vi "VCS Get Device Name.vi"(8 "error in (no error)":errorcluster, 11 "axis in":cluster{"keyHandle":u32, "nodeId":u16}={"keyHandle"=0, "nodeId"=1}) -> (0 "error out":errorcluster, 2 "deviceName":string, 3 "axis out":cluster{"keyHandle":u32, "nodeId":u16}={"keyHandle"=0, "nodeId"=1})   [LabVIEW 2019]
doc: "<B>VCS Get Device Name</B> returns the device name to corresponding handle."
uses:
  Resources/EposCmd.dll
  Examples/maxonEPOS.lvlib
  Resources/EposCmd64.dll
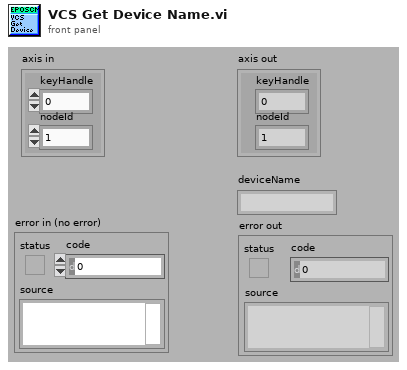
[diagram p1: front panel]
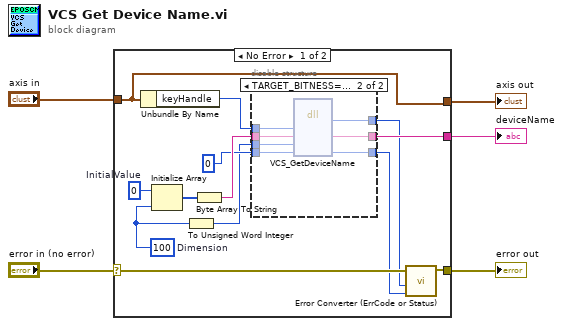
[diagram p0: block diagram]
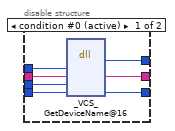
[diagram p2: hidden frame]
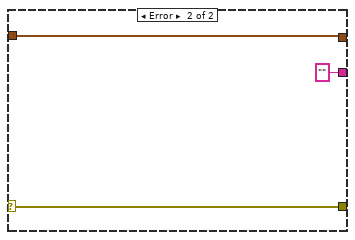
[diagram p3: hidden frame]
diagram:
  n1 = case shown="No Error" "error in (no error)" {
    selector: "error in (no error)" -> [w17 w35]
    tunnel: [w16 w35] -> w4
    tunnel: [w18 "" ("pDeviceName")] -> w3
    tunnel: "axis in" -> [w9 w34]
    tunnel: [w9 w34] -> w1
    frame No Error {
      w12 = u8 0  # InitialValue
      w6 = 100  # Dimension
      n2 = Unbundle By Name(w9) -> ("keyHandle"=w14:u32)
      n3 = Initialize Array(w12, w6) -> (w13:u8[])
      n4 = To Unsigned Word Integer(number=w6) -> (unsigned 16bit integer=w7:u16)
      n5 = Byte Array To String(unsigned byte array=w13) -> (string=w11:string)
      n6 = disable-structure shown="TARGET_BITNESS==64" {
        disable-tunnel: [w25 w32] -> w18
        disable-tunnel: [w24 w31] -> w15
        disable-tunnel: w14 -> [w23 w30]
        disable-tunnel: w11 -> [w22 w29]
        disable-tunnel: u32 0 ("pErrorCode") -> [w21 w28]
        disable-tunnel: [w20 w27] -> w8
        disable-tunnel: w7 -> [w19 w26]
        frame condition #0 (active) {
          n7 = dll-call lib="C:/workspace/project/scancon/sw/SSI_Tool/InstrumentsInterfaces/Motordriver/maxon EPOS/Resources/EposCmd.*" fn="_VCS_GetDeviceName@16"("KeyHandle"=w23, "pDeviceName"=w22, "MaxStrSize"=w19, "pErrorCode"=w21) -> (w20:i32, "pDeviceName"=w25:string, "pErrorCode"=w24:u32)  [unwired: 5 in, 2 out]
        }
        frame condition #1 {
          n8 = dll-call lib="C:/Sources/LabView/maxon EPOS/Resources/EposCmd64.*" fn="VCS_GetDeviceName" ("EposCmd.dll:_VCS_GetDeviceName@16")("KeyHandle"=w30, "pDeviceName"=w29, "MaxStrSize"=w26, "pErrorCode"=w28) -> ("Rückgabetyp"=w27:i32, "pDeviceName"=w32:string, "pErrorCode"=w31:u32)  [unwired: 5 in, 2 out]
        }
      }
      n9 = call "Error Converter (ErrCode or Status).vi"("error code"=w15, "return type"=w8, "error in (no error)"=w17) -> ("error out"=w16:errorcluster)  [unwired: 7 in]
    }
    frame Error {
    }
  }
  "deviceName" <- w3
  "error out" <- w4
  "axis out" <- w1
